vi "CRYSet Recnent Menu.vi"(10 "menuc tag":string, 11 "Main Menu Refnum in":refnum<k9>) -> (3 "Main Menu Refnum out":refnum<k9>)   [LabVIEW 2013]
uses:
  CRYMainGlobal.vi
panel:
  # "Set recent menu."
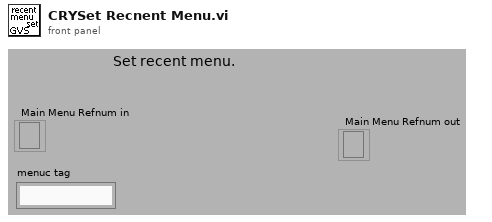
[diagram p1: front panel]
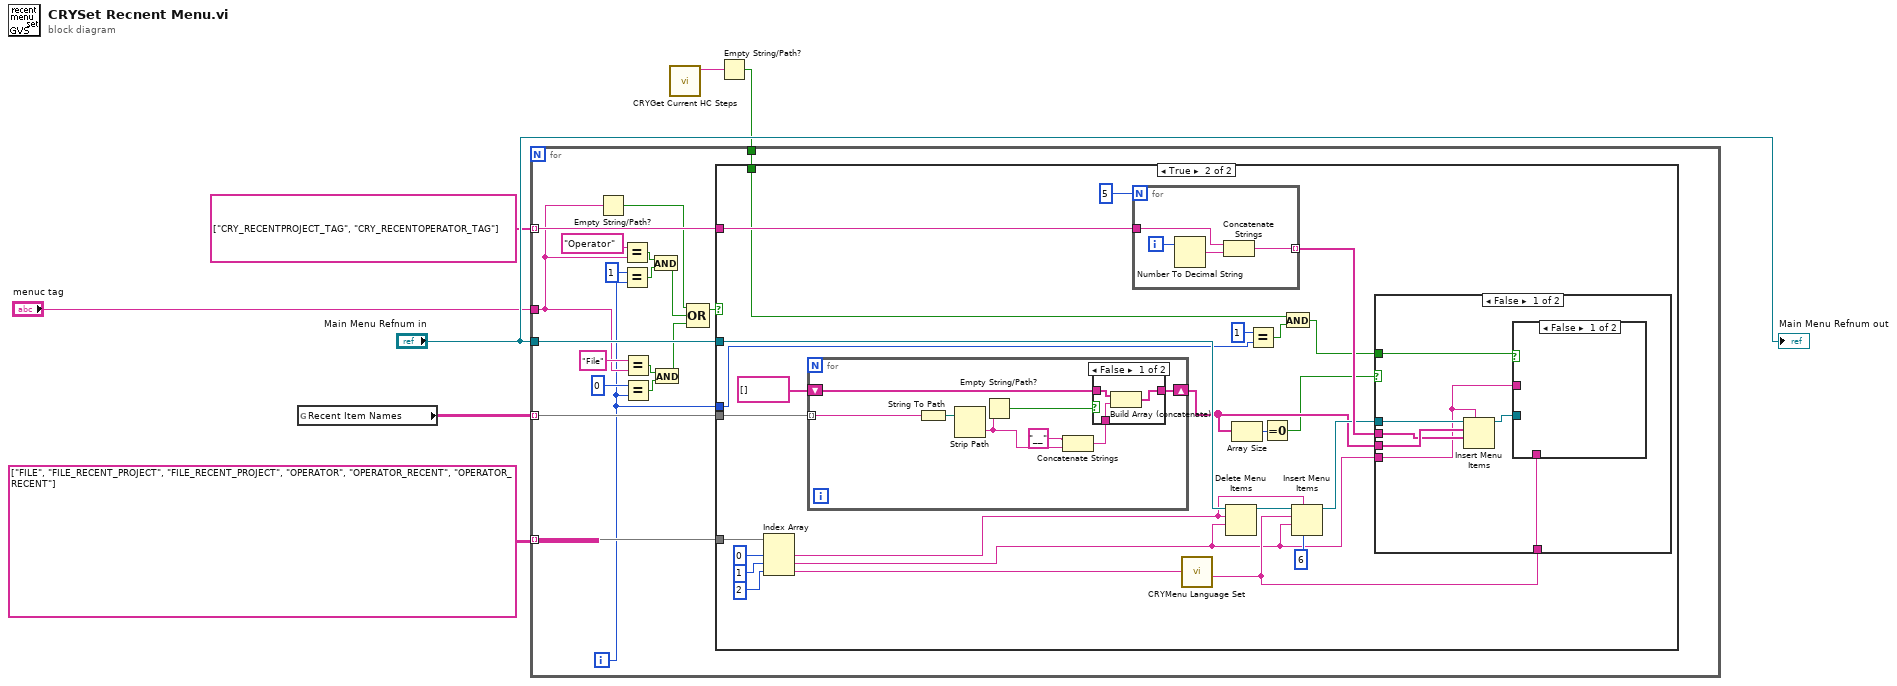
[diagram p0: block diagram]
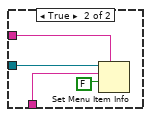
[diagram p4: hidden frame]
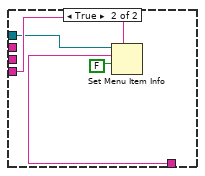
[diagram p5: hidden frame]
diagram:
  n1 = global read "CRYMainGlobal.vi" "Recent Item Names"() -> (w4:string[][])
  n2 = call "CRYGet Current HC Steps.vi"() -> ("Hardware setup flattened Out"=w2:string)  [unwired: 10 in, 1 out]
  n3 = Empty String/Path?(string/path=w2) -> (empty?=w1:bool)
  n4 = for {
    tunnel: w4 -> [w26] mode=indexing
    tunnel: "Main Menu Refnum in" -> [w25]
    tunnel: string[] ["CRY_RECENTPROJECT_TAG", "CRY_RECENTOPERATOR_TAG"] -> [w24] mode=indexing
    tunnel: string[][] [["FILE", "FILE_RECENT_PROJECT", "FILE_RECENT_PROJECT"], ["OPERATOR", "OPERATOR_RECENT", "OPERATOR_RECENT"]] -> [w23] mode=indexing
    tunnel: "menuc tag" -> [w11]
    tunnel: w1 -> [w8]
    i -> [w9]
    n5 = Empty String/Path?(string/path=w11) -> (empty?=w12:bool)
    n6 = Equal?(x="Operator" ("y"), y=w11) -> (x = y?=w21:bool)
    n7 = Equal?(x=1, y=w9) -> (x = y?=w20:bool)
    n8 = Equal?(x="File" ("y"), y=w11) -> (x = y?=w16:bool)
    n9 = Equal?(x=0, y=w9) -> (x = y?=w17:bool)
    n10 = And(x=w21, y=w20) -> (x .and. y?=w19:bool)
    n11 = And(x=w16, y=w17) -> (x .and. y?=w13:bool)
    n12 = Compound Arithmetic op=OR(w12, w19, w13) -> (w18:bool)
    n13 = case shown="True" w18 {
      tunnel: w26 -> [_ w27]
      tunnel: w25 -> [_ w46]
      tunnel: w24 -> [_ w43]
      tunnel: w23 -> [_ w42]
      tunnel: w9 -> [_ w32]
      tunnel: w8 -> [_ w30]
      frame False {
      }
      frame True {
        n14 = Index Array(array=w42, index #1=0 ("index"), index #2=1 ("index"), index #3=2 ("index")) -> (element #1=w41:string, element #2=w40:string, element #3=w39:string)
        n15 = for {
          tunnel: w27 -> [w55] mode=indexing
          shift-right: [w56] -> w34
          shift-left: string[] [] -> [w57]
          n16 = String To Path(string=w55) -> (path=w59:path)
          n17 = Strip Path(path=w59) -> (name=w53:string)  [unwired: 1 out]
          n18 = Empty String/Path?(string/path=w53) -> (empty?=w58:bool)
          n19 = Concatenate Strings("__", w53) -> (w54:string)
          n20 = case shown="False" w58 {
            tunnel: w57 -> [w62 w63]
            tunnel: [w61 w63] -> w56
            tunnel: w54 -> [w60 _]
            frame False {
              n21 = Build Array (concatenate)(w62, w60) -> (w61:string[])
            }
            frame True {
            }
          }
        }
        n22 = for {
          N: 5 -> [_]
          tunnel: [w80] -> w49 mode=indexing
          tunnel: w43 -> [w79]
          i -> [w82]
          n23 = Number To Decimal String(number=w82) -> (decimal integer string=w81:string)  [unwired: 1 out]
          n24 = Concatenate Strings(w79, w81) -> (w80:string)
        }
        n25 = call "CRYMenu Language Set.vi"("sID"=w39) -> ("sMultibyte_Out"=w44:string)  [unwired: 7 in, 3 out]
        n26 = Delete Menu Items(7:w40, 8:w41, 9:w46) -> (3:w48:refnum<k9>)  [unwired: 1 in, 1 out]
        n27 = Array Size(array=w34) -> (size(s)=w50:i32)
        n28 = Equal?(x=1, y=w32) -> (x = y?=w31:bool)
        n29 = Equal To 0?(x=w50) -> (x = 0?=w29:bool)
        n30 = And(x=w30, y=w31) -> (x .and. y?=w28:bool)
        n31 = Insert Menu Items(4:6 ("y"), 5:w41, 7:w40, 8:w44, 9:w48) -> (3:w45:refnum<k9>)  [unwired: 1 in, 2 out]
        n32 = case shown="False" w29 {
          tunnel: w40 -> [w66 w78]
          tunnel: w34 -> [w70 _]
          tunnel: w49 -> [w69 _]
          tunnel: w45 -> [w68 w76]
          tunnel: w44 -> [w65 w75]
          tunnel: w28 -> [w64 _]
          frame False {
            n33 = Insert Menu Items(5:w66, 7:w69, 8:w70, 9:w68) -> (3:w67:refnum<k9>)  [unwired: 1 in, 3 out]
            n34 = case shown="False" w64 {
              tunnel: w67 -> [_ w73]
              tunnel: w66 -> [_ w72]
              tunnel: w65 -> [_ w71]
              frame False {
              }
              frame True {
                n35 = Set Menu Item Info(7:w72, 9:FALSE ("enabled"), 10:w71, 11:w73) -> ()  [unwired: 1 in, 4 out]
              }
            }
          }
          frame True {
            n36 = Set Menu Item Info(7:w78, 9:FALSE ("enabled"), 10:w75, 11:w76) -> ()  [unwired: 1 in, 4 out]
          }
        }
      }
    }
  }
  "Main Menu Refnum out" <- "Main Menu Refnum in"
